vi "Get Client Certificate (Client).vi"(10 "Client Certificates":T1) -> (2 "client certificate file":path)   [LabVIEW 2014, in "OPC UA Client runtime.lvclass"]
doc: "Get client certificate used to create an OPC UA client connection"
uses:
  OPC UA Client runtime.lvclass
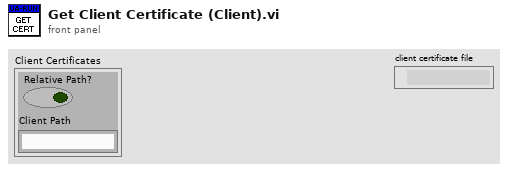
[diagram p1: front panel]
types:
  T1 = cluster{"Relative Path?":bool, "Client Path":string}
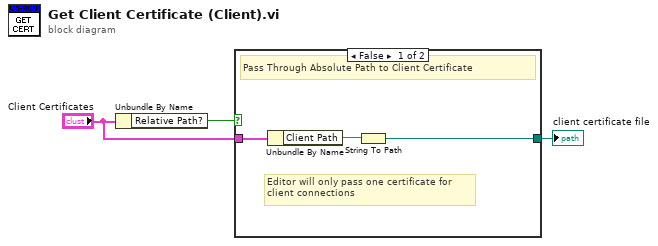
[diagram p0: block diagram]
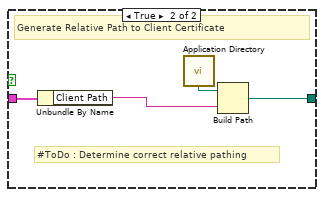
[diagram p2: hidden frame]
diagram:
  n1 = Unbundle By Name("Client Certificates") -> ("Relative Path?"=w3:bool)
  n2 = case shown="False" w3 {
    tunnel: "Client Certificates" -> [w6 w10]
    tunnel: [w4 w8] -> w1
    frame False {
      # "Editor will only pass one certificate for\nclient connections"
      # "Pass Through Absolute Path to Client Certificate"
      n3 = Unbundle By Name(w6) -> ("Client Path"=w5:string)
      n4 = String To Path(string=w5) -> (path=w4:path)
    }
    frame True {
      # "#ToDo : Determine correct relative pathing"
      # "Generate Relative Path to Client Certificate"
      n5 = Unbundle By Name(w10) -> ("Client Path"=w7:string)
      n6 = call <vilib>:"Application Directory.vi"() -> ("Application Directory"=w9:path)
      n7 = Build Path(base path=w9, name or relative path=w7) -> (appended path=w8:path)
    }
  }
  "client certificate file" <- w1
